vi "xwpfDocument Tests Write.vi"   [LabVIEW 2017, in "Word_Specific.lvlib"]
uses:
  src/LabVIEW NPOI/Word_Specific.lvlib
  src/LabVIEW NPOI/xwpfDocument/xwpfDocument.lvclass
types:
  T1 = enum16{"Title", "Heading 1", "Heading 2", "Heading 3", "Normal", "Figure", "Page Break"}[]
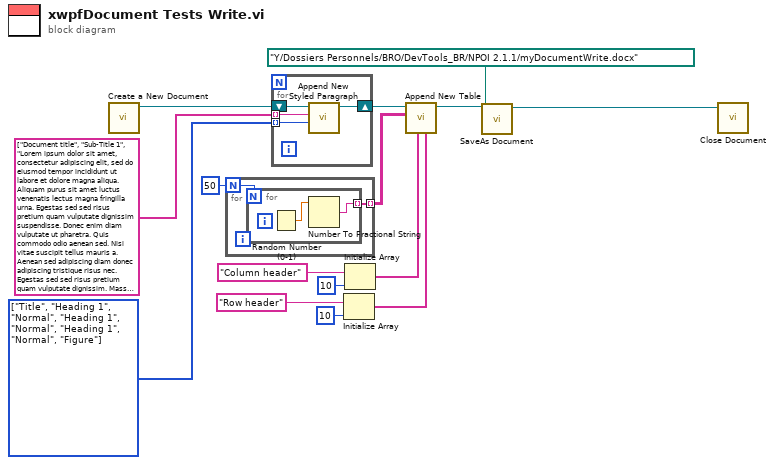
[diagram p0: block diagram]
diagram:
  w13 = T1 [enum."Title", enum."Heading 1", enum."Normal", enum."Heading 1", enum."Normal", enum."Heading 1", enum."Normal", enum."Figure"] items=["Title", "Heading 1", "Heading 2", "Heading 3", "Normal", "Figure", "Page Break"]
  n1 = call "Create a New Document.vi"() -> ("xwpfDocument out"=w12:refnum<class "xwpfDocument.lvclass">)  [unwired: 10 in, 1 out]
  n2 = for {
    N: 50 -> [w16]
    tunnel: [w17] -> w7 mode=indexing
    n3 = for {
      N: w16 -> [_]
      tunnel: [w18] -> w17 mode=indexing
      n4 = Random Number (0-1)() -> (number: 0 to 1=w19:dbl)
      n5 = Number To Fractional String(number=w19) -> (F-format string=w18:string)  [unwired: 3 in]
    }
  }
  n6 = for {
    shift-right: [w22] -> w10
    shift-left: w12 -> [w23]
    tunnel: string[] ["Document title", "Sub-Title 1", "Lorem ipsum dolor sit amet, consectetur adipiscing elit, sed do eiusmod tempor incididunt ut labore et dolore magna aliqua. Aliquam purus sit amet luctus venenatis lectus magna fringilla urna. Egestas sed sed risus pretium quam vulputate dignissim suspendisse. Donec enim diam vulputate ut pharetra. Quis commodo odio aenean sed. Nisi vitae suscipit tellus mauris a. Aenean sed adipiscing diam donec adipiscing tristique risus nec. Egestas sed sed risus pretium quam vulputate dignissim. Massa placerat duis ultricies lacus. Nec feugiat nisl pretium fusce id velit ut tortor pretium. Tincidunt tortor aliquam nulla facilisi cras fermentum odio eu feugiat. Feugiat sed lectus vestibulum mattis ullamcorper velit sed ullamcorper. Pulvinar mattis nunc sed blandit libero volutpat. Pulvinar elementum integer enim neque volutpat ac tincidunt vitae.", "Sub-Title 2", "Lorem ipsum dolor sit amet, consectetur adipiscing elit, sed do eiusmod tempor incididunt ut labore et dolore magna aliqua. Aliquam purus sit amet luctus venenatis lectus magna fringilla urna. Egestas sed sed risus pretium quam vulputate dignissim suspendisse. Donec enim diam vulputate ut pharetra. Quis commodo odio aenean sed. Nisi vitae suscipit tellus mauris a. Aenean sed adipiscing diam donec adipiscing tristique risus nec. Egestas sed sed risus pretium quam vulputate dignissim. Massa placerat duis ultricies lacus. Nec feugiat nisl pretium fusce id velit ut tortor pretium. Tincidunt tortor aliquam nulla facilisi cras fermentum odio eu feugiat. Feugiat sed lectus vestibulum mattis ullamcorper velit sed ullamcorper. Pulvinar mattis nunc sed blandit libero volutpat. Pulvinar elementum integer enim neque volutpat ac tincidunt vitae.", "Sub-Title 3", "Lorem ipsum dolor sit amet, consectetur adipiscing elit, sed do eiusmod tempor incididunt ut labore et dolore magna aliqua. Aliquam purus sit amet luctus venenatis lectus magna fringilla urna. Egestas sed sed risus pretium quam vulputate dignissim suspendisse. Donec enim diam vulputate ut pharetra. Quis commodo odio aenean sed. Nisi vitae suscipit tellus mauris a. Aenean sed adipiscing diam donec adipiscing tristique risus nec. Egestas sed sed risus pretium quam vulputate dignissim. Massa placerat duis ultricies lacus. Nec feugiat nisl pretium fusce id velit ut tortor pretium. Tincidunt tortor aliquam nulla facilisi cras fermentum odio eu feugiat. Feugiat sed lectus vestibulum mattis ullamcorper velit sed ullamcorper. Pulvinar mattis nunc sed blandit libero volutpat. Pulvinar elementum integer enim neque volutpat ac tincidunt vitae.", "C:\\Users\\Neo\\Desktop\\Dev_Tools_BR\\LabVIEW_NPOI\\tests\\Test Cases\\image.png"] -> [w21] mode=indexing
    tunnel: w13 -> [w20] mode=indexing
    n7 = call "Append New Styled Paragraph.vi"("Type"=w20, "Paragraph.Text"=w21, "xwpfDocument in"=w23) -> ("xwpfDocument out"=w22:refnum<class "xwpfDocument.lvclass">)  [unwired: 7 in, 1 out]
  }
  n8 = Initialize Array("Row header", 10 ("dimension size")) -> (w1:string[])
  n9 = Initialize Array("Column header", 10 ("dimension size")) -> (w4:string[])
  n10 = call "Append New Table.vi"("Row.Headers"=w1, "Column.Headers"=w4, "Table.Data"=w7, "xwpfDocument in"=w10) -> ("xwpfDocument out"=w9:refnum<class "xwpfDocument.lvclass">)  [unwired: 6 in, 1 out]
  n11 = call "SaveAs Document.vi"("Document Path"=path "Y:/Dossiers Personnels/BRO/DevTools_BR/NPOI 2.1.1/myDocumentWrite.docx", "xwpfDocument in"=w9) -> ("xwpfDocument out"=w15:refnum<class "xwpfDocument.lvclass">)  [unwired: 8 in, 1 out]
  n12 = call "Close Document.vi"("xwpfDocument in"=w15) -> ()  [unwired: 9 in, 2 out]
